vi "Populate Plot Data Array with Shared Variable Data.vi"(8 "error in":errorcluster, 10 "Plot Channel Configurations":T1[](array[typedef]), 11 "Plot Data In":T2[](array[typedef])) -> (0 "error out":errorcluster, 1 "Update Timestamps":timestamp[](array[timestamp]), 2 "Data Updated":bool[](array[boolean]), 3 "Plot Data Out":T2[](array[typedef]))   [LabVIEW 2017, in "DTacq Plot Display Library.lvlib"]
doc: "Reads shared variable values, and puts the data into the plot data array.\n\nNote, the for loop itterates over the smaller array. When array sizes change, this can\ncause old data to reamain stored in the plot."
uses:
  DTacq Plot Display Library.lvlib
  Plot Data--Cluster.ctl
  Network Shared Variables/Typedefs/X and Y Variant Arrays--Cluster.ctl
  Typedefs/Plot Channel Configruation--Cluster.ctl
  Network Shared Variables/Shared Variables Library.lvlib
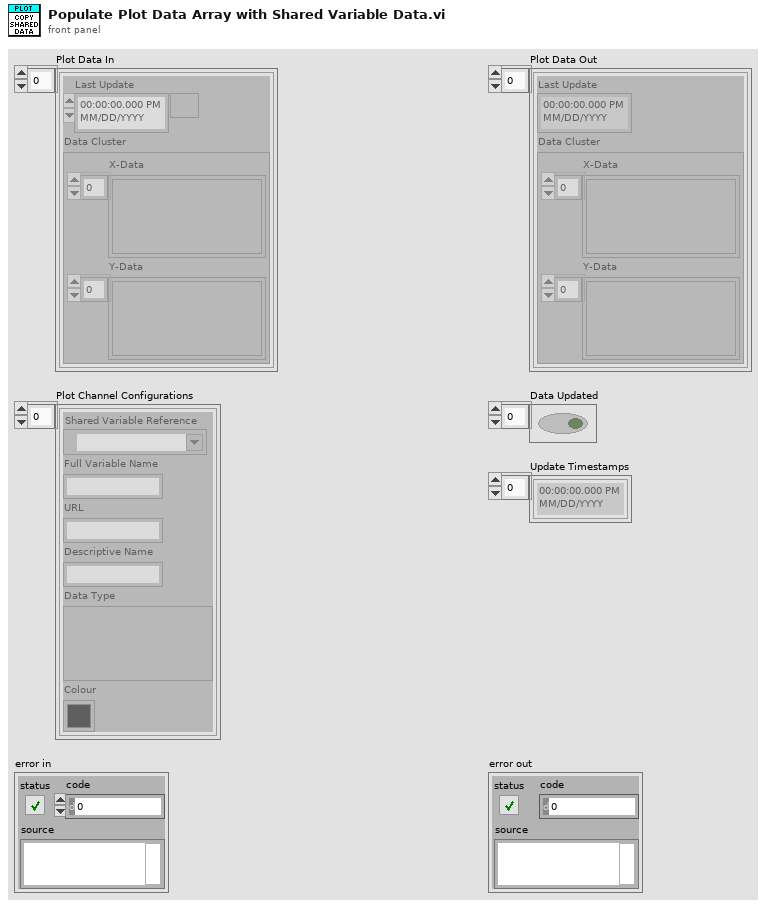
[diagram p1: front panel]
types:
  T1 = typedef "DTacq Plot Display Library.lvlib/Plot Channel Configruation--Cluster.ctl" = cluster{"Shared Variable Reference":refnum<k21>, "Full Variable Name":string, "URL":string, "Descriptive Name":string, "Data Type":variant, "Colour":u32}
  T2 = typedef "DTacq Plot Display Library.lvlib/Plot Data--Cluster.ctl" = cluster{"Last Update":timestamp, "Data Cluster":T3}
  T3 = typedef "Shared Variables Library.lvlib/X and Y Variant Arrays--Cluster.ctl" = cluster{"X-Data":variant[], "Y-Data":variant[]}
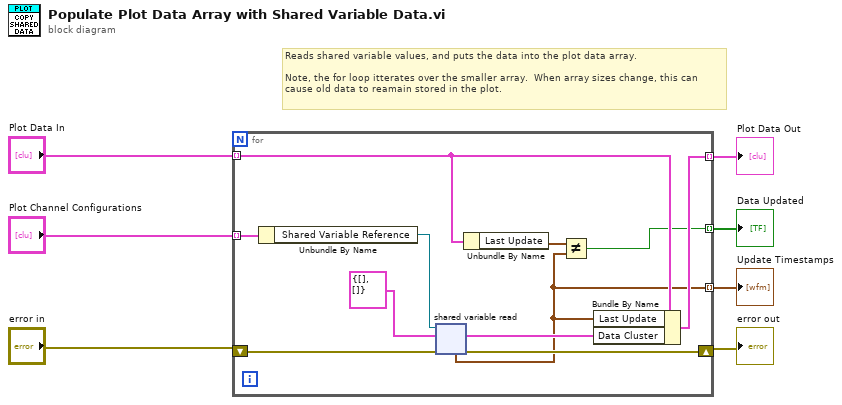
[diagram p0: block diagram]
diagram:
  # "Reads shared variable values, and puts the data into the plot data array.\n\nNote, the for loop itterates over the smaller array.  When array sizes change, this can\ncause old data to reamain stored in the plot."
  n1 = for {
    tunnel: "Plot Channel Configurations" -> [w18] mode=indexing
    shift-right: [w13] -> w3
    shift-left: "error in" -> [w17]
    tunnel: [w9] -> w4 mode=indexing
    tunnel: "Plot Data In" -> [w14] mode=indexing
    tunnel: [w11] -> w6 mode=indexing
    tunnel: [w8] -> w7 mode=indexing
    n2 = Unbundle By Name(w18) -> ("Shared Variable Reference"=w16:refnum<k21>)
    n3 = shared-variable-read(w16, w17, T3 {"X-Data"=[], "Y-Data"=[]} ("Data Cluster")) -> (w13:errorcluster, w12:T3, w8:timestamp)  [unwired: 1 out]
    n4 = Unbundle By Name(w14) -> ("Last Update"=w10:timestamp)
    n5 = Not Equal?(x=w10, y=w8) -> (x != y?=w9:bool)
    n6 = Bundle By Name(cluster=w14, "Last Update"=w8, "Data Cluster"=w12) -> (w11:T2)
  }
  "Update Timestamps" <- w7
  "Plot Data Out" <- w6
  "Data Updated" <- w4
  "error out" <- w3
